vi "baseline calculator.vi"(7 "method":i32(ring)=1 items=["median", "noise center", "Minimum", "lower 20th"], 10 "timetrace":dbl[](array[numeric])) -> (2 "baseline":dbl format="%0.2f")   [LabVIEW 2009]
uses:
  <vilib>/gmath/statdist.llb/st_Percentiles (scalar).vi
  <vilib>/Analysis/NI_AALBase.lvlib
  <vilib>/gmath/NI_Gmath.lvlib
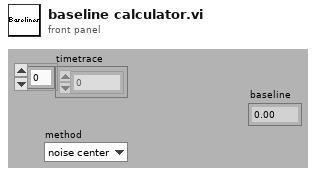
[diagram p1: front panel]
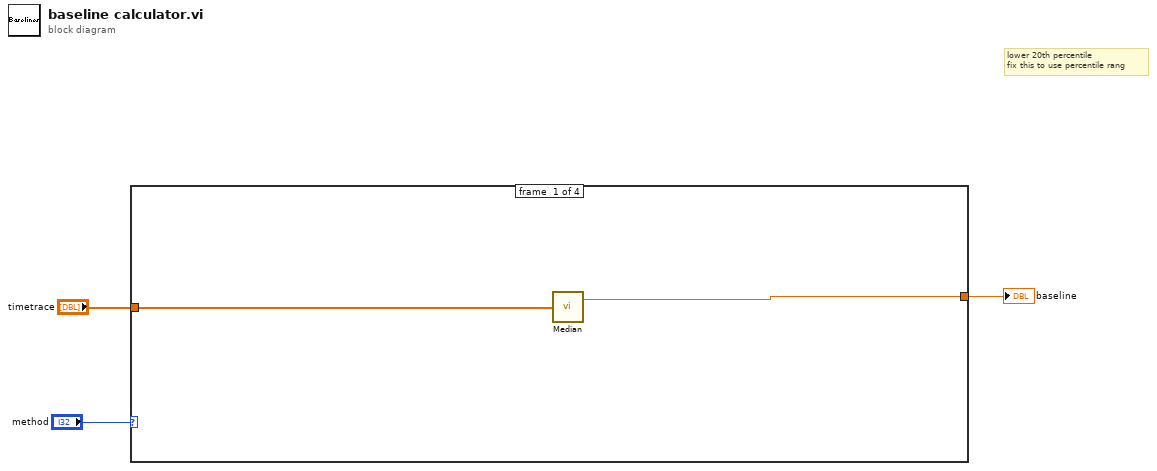
[diagram p0: block diagram]
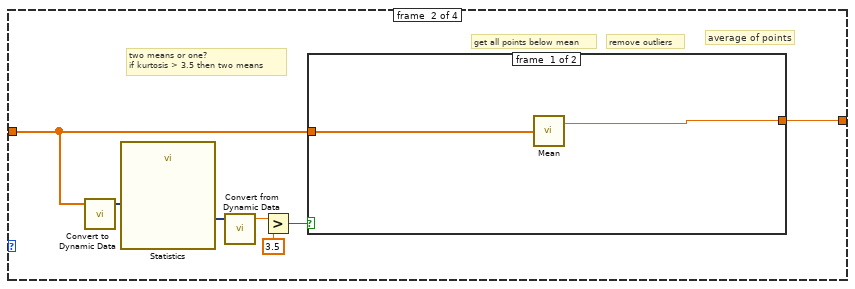
[diagram p2: hidden frame]
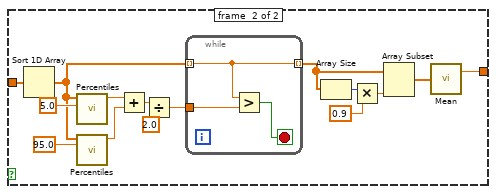
[diagram p3: hidden frame]
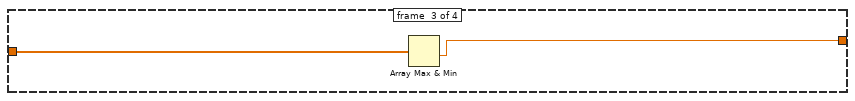
[diagram p4: hidden frame]
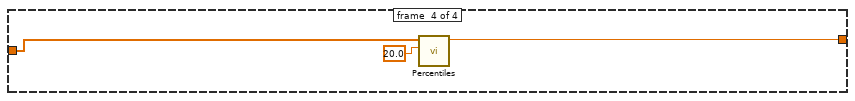
[diagram p5: hidden frame]
diagram:
  # "lower 20th percentile\nfix this to use percentile rang"
  n1 = case shown="3" "method" {
    tunnel: "timetrace" -> [w5 w7 w34 w37]
    tunnel: [w4 w6 w33 w36] -> w1
    frame #0 {
      n2 = call <vilib>:"Median.vi"("X"=w5) -> ("median"=w4:dbl)  [unwired: 1 out]
    }
    frame #1 {
      # "remove outliers"
      # "average of points"
      # "two means or one?\nif kurtosis > 3.5 then two means"
      # "get all points below mean"
      n3 = call "Convert to Dynamic Data"("Array"=w7) -> ("Dynamic Data Type"=w12:dynamicdata)  [unwired: 3 in]
      n4 = call "Statistics"("Signals"=w12) -> ("Kurtosis"=w11:dynamicdata)  [unwired: 24 in, 2 out]
      n5 = call "Convert from Dynamic Data"("Dynamic Data Type"=w11) -> ("Scalar"=w8:dbl)  [unwired: 3 in]
      n6 = Greater?(x=w8, y=3.5) -> (0:w9:bool)
      n7 = case shown="True" w9 {
        tunnel: w7 -> [w14 w29]
        tunnel: [w13 w22] -> w6
        frame #0 {
          n8 = call <vilib>:"Mean.vi"("X"=w14) -> ("mean"=w13:dbl)  [unwired: 1 out]
        }
        frame #1 {
          n9 = Sort 1D Array(array=w29) -> (sorted array=w20:dbl[])
          n10 = call-poly <vilib>:"Percentiles.vi"("p"=5.0, "x array"=w20) -> ("percentile"=w17:dbl)  [unwired: 8 in, 1 out]
          n11 = call-poly <vilib>:"Percentiles.vi"("p"=95.0, "x array"=w20) -> ("percentile"=w16:dbl)  [unwired: 8 in, 1 out]
          n12 = Add(x=w17, y=w16) -> (x+y=w15:dbl)
          n13 = Divide(x=w15, y=2.0) -> (x/y=w18:dbl)
          n14 = while {
            tunnel: w20 -> [w31] mode=indexing
            tunnel: [w31] -> w25 mode=indexing
            tunnel: w18 -> [w30]
            stop <- w32 stop-if-true
            n15 = Greater?(x=w31, y=w30) -> (0:w32:bool)
          }
          n16 = Array Size(array=w25) -> (size(s)=w28:i32)
          n17 = Multiply(x=w28, y=0.9) -> (x*y=w26:dbl)
          n18 = Array Subset(array=w25, length=w26) -> (w24:dbl[])  [unwired: 1 in]
          n19 = call <vilib>:"Mean.vi"("X"=w24) -> ("mean"=w22:dbl)  [unwired: 1 out]
        }
      }
    }
    frame #2 {
      n20 = Array Max & Min(array=w34) -> (min value=w33:dbl)  [unwired: 3 out]
    }
    frame #3 {
      n21 = call-poly <vilib>:"Percentiles.vi"("p"=20.0, "x array"=w37) -> ("percentile"=w36:dbl)  [unwired: 8 in, 1 out]
    }
  }
  "baseline" <- w1
